vi "Read Spectral Calibration.vi"(11 "Analyze Parameter Spectral Calibration in":refnum<class "Analyze Parameter Spectral Calibration.lvclass">) -> (0 "Central WL":dbl[unit], 1 "Central Pixel":i32, 2 "nm per px":dbl[unit], 3 "Analyze Parameter Spectral Calibration out":refnum<class "Analyze Parameter Spectral Calibration.lvclass">)   [LabVIEW 2014, in "Analyze Parameter Spectral Calibration.lvclass"]
uses:
  Analyze Parameter Spectral Calibration.lvclass
  Analyze Parameter Spectral Calibration.lvclass/Analyze Parameter Spectral Calibration.ctl
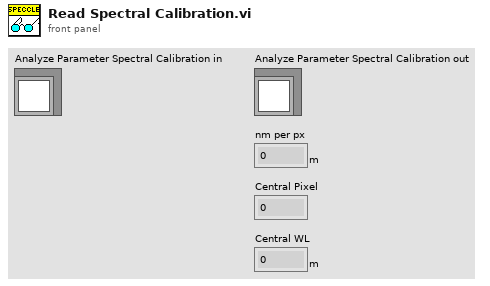
[diagram p1: front panel]
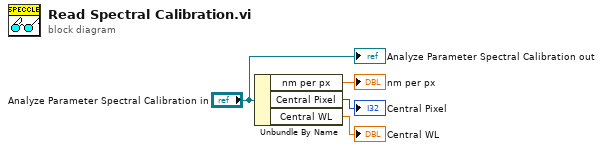
[diagram p0: block diagram]
diagram:
  n1 = Unbundle By Name("Analyze Parameter Spectral Calibration in") -> ("nm per px"=→"nm per px":dbl[unit], "Central Pixel"=→"Central Pixel":i32, "Central WL"=→"Central WL":dbl[unit])
  "Analyze Parameter Spectral Calibration out" <- "Analyze Parameter Spectral Calibration in"
